vi "Init.vi"(8 "error in (no error)":errorcluster, 10 "Event Subs (All)":T1[](array[typedef]) items=["None"=0, "General"=1, "Config"=2, "Scenes"=4, "Inputs"=8, "Transitions"=16, "Filters"=32, "Outputs"=64, "SceneItems"=128, "MediaInputs"=256, "Vendors"=512, "UI"=1024, "NonHighVolume"=1023, "InputVolumeMeters"=65536, "InputActiveStateChanged"=131072, "InputShowStateChanged"=262144, "SceneItemTransformChanged"=524288], 11 "RPC Version":i32) -> (0 "error out":errorcluster, 3 "Identify out":refnum<class "Identify.lvclass">)   [LabVIEW 2022 SP3, in "obs-websocket-lv.lvlib" / "Identify.lvclass"]
uses:
  Identify.lvclass
  Identify.lvclass/Identify.ctl
  Event Subscription.ctl
  obs-websocket-lv.lvlib
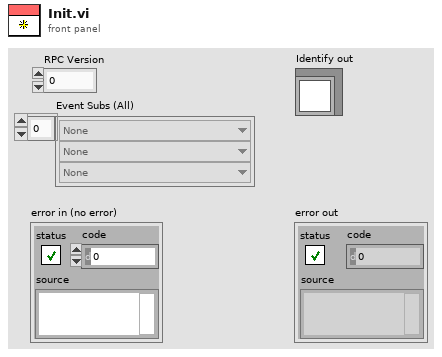
[diagram p1: front panel]
types:
  T1 = typedef "obs-websocket-lv.lvlib/Event Subscription.ctl" = u32
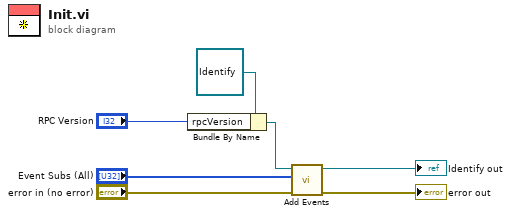
[diagram p0: block diagram]
diagram:
  n1 = Bundle By Name(cluster=refnum<class "Identify.lvclass"> refnum ("Identify in"), "rpcVersion"="RPC Version") -> (w1:refnum<class "Identify.lvclass">)
  n2 = call "Add Events.vi"("error in (no error)"="error in (no error)", "Event Subs (All)"="Event Subs (All)", "Identify in"=w1) -> ("error out"=→"error out":errorcluster, "Identify out"=→"Identify out":refnum<class "Identify.lvclass">)  [unwired: 7 in]
